vi "Read TCPIP address.vi"(8 "error in (no error)":errorcluster, 11 "ESP301viaTCPIP in":refnum<class "ESP301viaTCPIP.lvclass">) -> (0 "error out":errorcluster, 2 "TCPIP address":string, 3 "ESP301viaTCPIP out":refnum<class "ESP301viaTCPIP.lvclass">)   [LabVIEW 2019, in "ESP301viaTCPIP.lvlib" / "ESP301viaTCPIP.lvclass"]
uses:
  ESP301viaTCPIP.lvclass
  ESP301viaTCPIP.lvclass/ESP301viaTCPIP.ctl
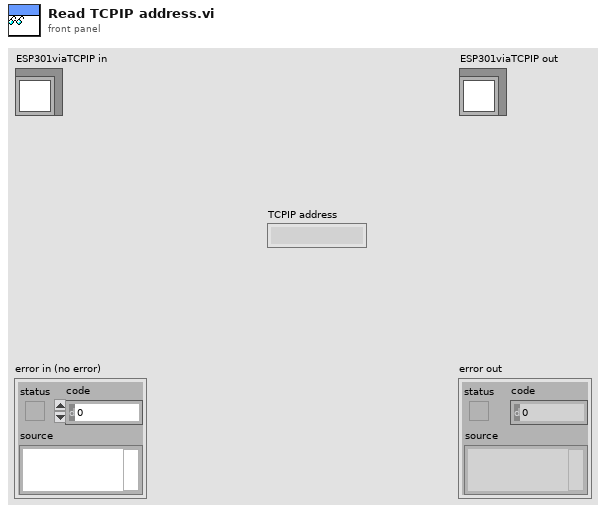
[diagram p1: front panel]
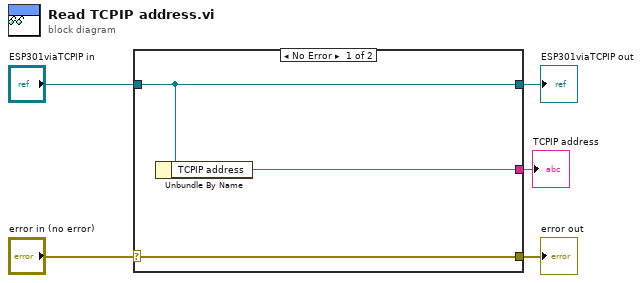
[diagram p0: block diagram]
diagram:
  n1 = case shown="No Error" "error in (no error)" {
    selector: "error in (no error)" -> [w8 w9]
    tunnel: [w8 w9] -> w4
    tunnel: [w7 w10] -> w2
    tunnel: "ESP301viaTCPIP in" -> [w7 w10]
    tunnel: [w6 _] -> w1
    frame No Error {
      n2 = Unbundle By Name(w7) -> ("TCPIP address"=w6:string)
    }
    frame Error {
    }
  }
  "error out" <- w4
  "ESP301viaTCPIP out" <- w2
  "TCPIP address" <- w1
